vi "Error Dialog.vi"(6 "Modal (T)":bool=TRUE, 8 "error in (no error)":errorcluster) -> (0 "error out":errorcluster)   [LabVIEW 2017, in "Error Dialog w Copy to Clipboard.lvlib"]
doc: "Displays error message to the user.\n\nCopyright (c) 2022, Neosoft Technologies Inc\nAll rights reserved."
uses:
  Error Dialog w Copy to Clipboard.lvlib
  <vilib>/Utility/error.llb/DialogType.ctl
  <vilib>/Platform/browser.llb/Open URL in Default Browser (string).vi
panel:
  out "String":string
  out "Error Code":string
  in  "Show details":bool
  in  "Google":bool
  in  "Copy":bool
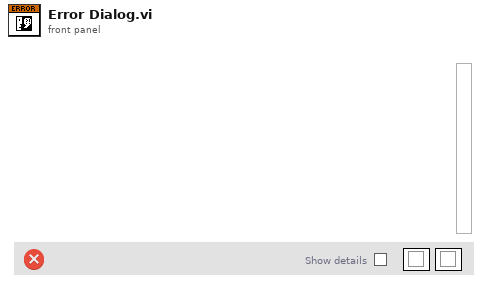
[diagram p1: front panel]
types:
  T1 = enum32{"Invalid", "Default", "Floating", "Floating/Auto-Hide", "Modal"}
  T2 = enum32{"Invalid", "Standard", "Closed", "Hidden", "Minimized", "Maximized"}
  T3 = cluster{"call chain":string[], "error":errorcluster, "show details":bool, "message":string}
  T4 = typedef "DialogType.ctl" = u16
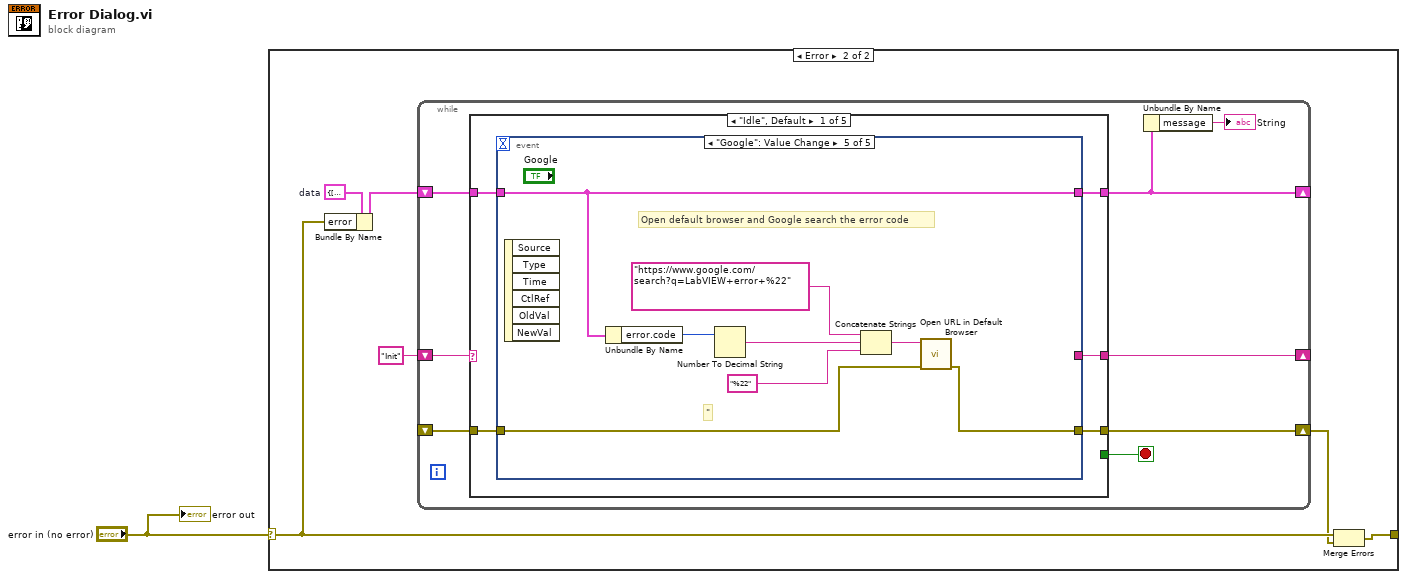
[diagram p0: block diagram]
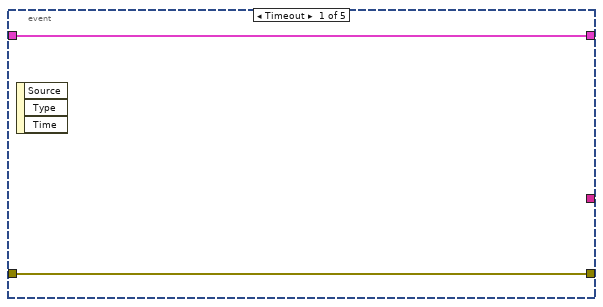
[diagram p3: hidden frame]
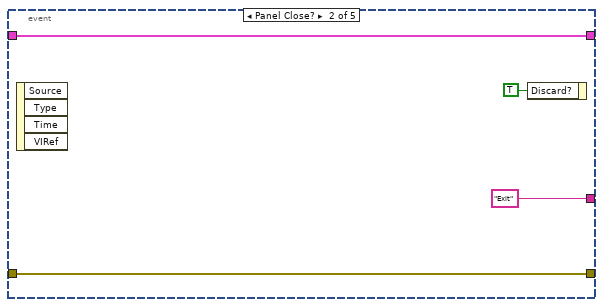
[diagram p4: hidden frame]
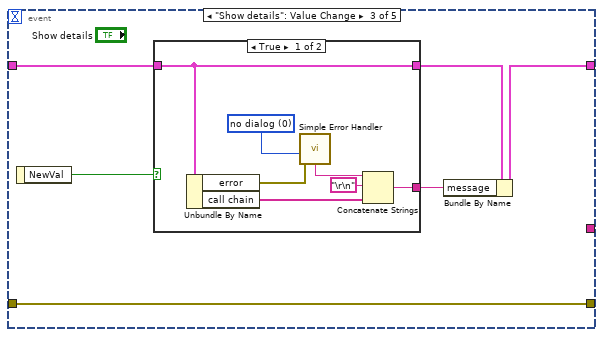
[diagram p5: hidden frame]
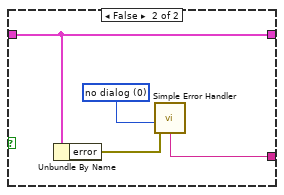
[diagram p6: hidden frame]
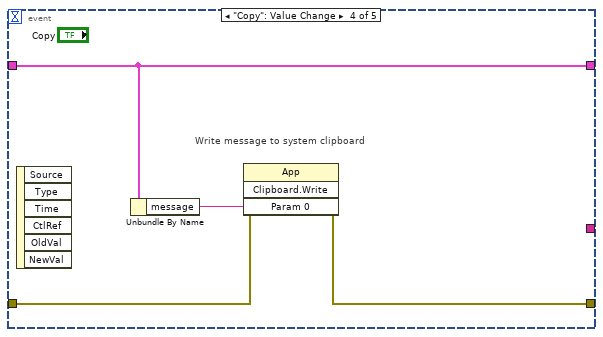
[diagram p7: hidden frame]
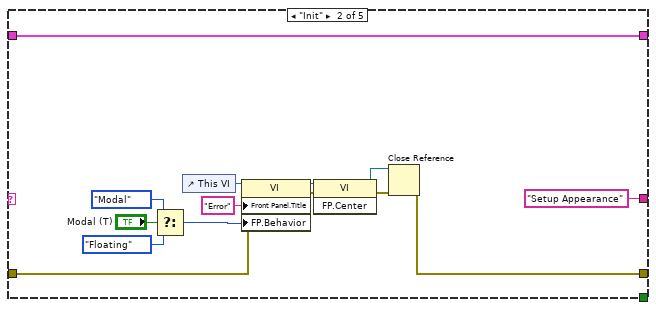
[diagram p8: hidden frame]
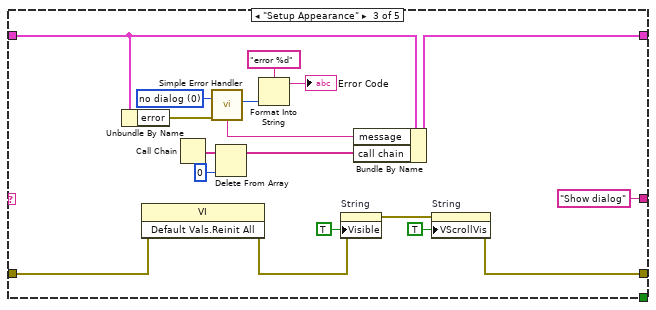
[diagram p9: hidden frame]
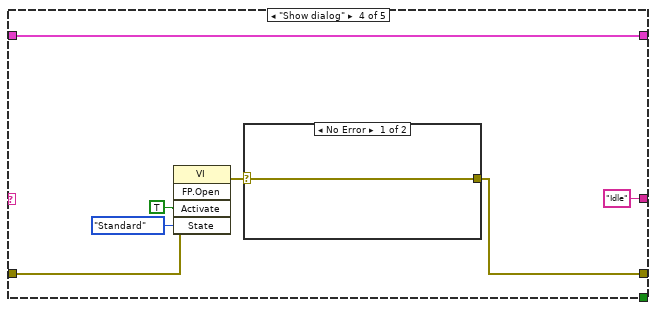
[diagram p10: hidden frame]
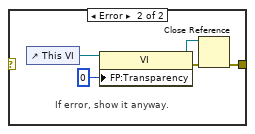
[diagram p11: hidden frame]
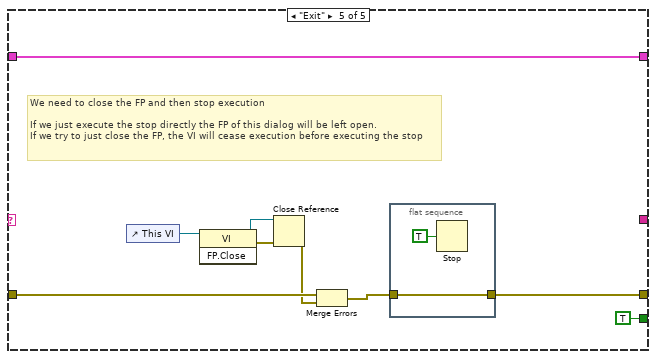
[diagram p12: hidden frame]
diagram:
  n1 = case shown="Error" "error in (no error)" {
    selector: "error in (no error)" -> [w2 w5]
    tunnel: [w2 w4] -> _
    frame No Error {
    }
    frame Error {
      w7 = T3 {"call chain"=[], "error"={"status"=FALSE, "code"=0, "source"=""}, "show details"=FALSE, "message"=""}  # data
      n2 = Bundle By Name(cluster=w7, "error"=w5) -> (w6:T3)
      n3 = while {
        shift-right: [w14] -> _
        shift-left: "Init" ("format string") -> [w15]
        shift-right: [w13] -> w3
        shift-left: _ -> [w12]
        shift-right: [w10] -> _
        shift-left: w6 -> [w11]
        stop <- w16 stop-if-true
        n4 = case shown="\"Idle\", Default" w15 {
          tunnel: [_ _ _ _ TRUE ("Discard?")] -> w16
          tunnel: [w17 "Setup Appearance" "Show dialog" "Idle" _] -> w14
          tunnel: [w20 w63 w79 w89 w104] -> w13
          tunnel: w12 -> [w21 w62 w72 w90 w110]
          tunnel: [w18 w61 w78 w95 w103] -> w10
          tunnel: w11 -> [w19 w61 w87 w95 w103]
          frame "Idle", Default {
            n5 = event shown="[4] \"Google\": Value Change" {
              selector: _ -> [_ _ _ _ _]
              dyn-events: _ -> [_ _ _ _ _]
              timeout: _ -> [_ _ _ _ _]
              tunnel: w21 -> [w23 w27 w33 w46 w54]
              tunnel: [w23 w27 w33 w45 w53] -> w20
              tunnel: w19 -> [w22 w26 w31 w48 w56]
              tunnel: [w22 w26 w29 w48 w56] -> w18
              tunnel: [_ "Exit" ("format string") _ _ _] -> w17
              event Timeout {
                n6 = event-data() -> ()  [unwired: 1 in, 3 out]
              }
              event Panel Close? {
                n7 = event-data() -> ()  [unwired: 1 in, 4 out]
                n8 = event-data("Discard?"=TRUE) -> ()  [unwired: 1 in, 1 out]
              }
              event "Show details": Value Change {
                n9 = event-data() -> ("NewVal"=w32:bool)  [unwired: 1 in]
                n10 = case shown="True" w32 {
                  tunnel: w31 -> [w38 w42]
                  tunnel: [w38 w42] -> w30
                  tunnel: [w34 w41] -> w28
                  frame True {
                    w37 = "\r\n"
                    w40 = T4 0 items=["no dialog", "OK message", "continue or stop message", "OK message + warnings", "continue/stop + warnings"] ("type of dialog (OK msg:1)")
                    n11 = Unbundle By Name(w38) -> ("error"=w39:errorcluster, "call chain"=w35:string[])
                    n12 = call <vilib>:"Simple Error Handler.vi"("type of dialog (OK msg:1)"=w40, "error in (no error)"=w39) -> ("message"=w36:string)  [unwired: 3 in, 4 out]
                    n13 = Concatenate Strings(w36, w37, w37, w35) -> (w34:string)
                  }
                  frame False {
                    w44 = T4 0 items=["no dialog", "OK message", "continue or stop message", "OK message + warnings", "continue/stop + warnings"] ("type of dialog (OK msg:1)")
                    n14 = Unbundle By Name(w42) -> ("error"=w43:errorcluster)
                    n15 = call <vilib>:"Simple Error Handler.vi"("type of dialog (OK msg:1)"=w44, "error in (no error)"=w43) -> ("message"=w41:string)  [unwired: 3 in, 4 out]
                  }
                }
                n16 = Bundle By Name(cluster=w30, "message"=w28) -> (w29:T3)
              }
              event "Copy": Value Change {
                # "Write message to system clipboard"
                n17 = event-data() -> ()  [unwired: 1 in, 6 out]
                n18 = Unbundle By Name(w48) -> ("message"=w47:string)
                n19 = invoke class="App" method="Clipboard.Write"(error in=w46, "Param 0"=w47) -> (error out=w45:errorcluster)  [unwired: 2 in, 3 out]
              }
              event "Google": Value Change {
                # "\""
                # "Open default browser and Google search the error code"
                n20 = event-data() -> ()  [unwired: 1 in, 6 out]
                n21 = Unbundle By Name(w56) -> ("error.code"=w50:i32)
                n22 = Number To Decimal String(number=w50) -> (decimal integer string=w49:string)  [unwired: 1 in]
                n23 = Concatenate Strings("https://www.google.com/search?q=LabVIEW+error+%22" ("format string"), w49, "%22") -> (w52:string)
                n24 = call-poly <vilib>:"Open URL in Default Browser.vi"("error in (no error)"=w54, "URL"=w52) -> ("error out"=w53:errorcluster)  [unwired: 4 in, 1 out]
              }
            }
          }
          frame "Init" {
            n25 = Select(t=T1."Modal" ("Front Panel Window:Behavior"), s="Modal (T)", f=T1."Floating") -> (s? t:f=w57:T1)
            n26 = control-ref of="This VI"() -> (w68:refnum<vi>)
            n27 = property class="VI"(reference=w68, error in=w62, "Front Panel.Title"="Error" ("Front Panel Window:Title"), "FP.Behavior"=w57) -> (reference out=w69:refnum<vi>, error out=w70:errorcluster)
            n28 = invoke class="VI" method="FP.Center"(reference=w69, error in=w70) -> (reference out=w66:refnum<vi>, error out=w65:errorcluster)  [unwired: 1 in, 1 out]
            n29 = Close Reference(reference=w66, error in (no error)=w65) -> (error out=w63:errorcluster)
          }
          frame "Setup Appearance" {
            w85 = T4 0 items=["no dialog", "OK message", "continue or stop message", "OK message + warnings", "continue/stop + warnings"] ("type of dialog (OK msg:1)")
            n30 = Unbundle By Name(w87) -> ("error"=w86:errorcluster)
            n31 = invoke class="VI" method="Default Vals.Reinit All"(error in=w72) -> (error out=w71:errorcluster)  [unwired: 2 in, 2 out]
            n32 = Call Chain() -> (call chain=w75:string[])
            n33 = call <vilib>:"Simple Error Handler.vi"("type of dialog (OK msg:1)"=w85, "error in (no error)"=w86) -> ("code out"=w84:i32, "message"=w77:string)  [unwired: 3 in, 3 out]
            n34 = Delete From Array(array=w75, index=0) -> (array with subset deleted=w74:string[])  [unwired: 1 in, 1 out]
            n35 = Format Into String(format string="error %d", w84) -> (resulting string=→"Error Code":string)  [unwired: 2 in, 1 out]
            n36 = property on="String" class="Str"(error in=w71, "Visible"=TRUE) -> (error out=w81:errorcluster)  [unwired: 1 in, 1 out]
            n37 = Bundle By Name(cluster=w87, "message"=w77, "call chain"=w74) -> (w78:T3)
            n38 = property on="String" class="Str"(error in=w81, "VScrollVis"=TRUE ("Vertical Scrollbar Visible")) -> (error out=w79:errorcluster)  [unwired: 1 in, 1 out]
          }
          frame "Show dialog" {
            n39 = invoke class="VI" method="FP.Open"(error in=w90, "Activate"=TRUE ("Front Panel Window:Open"), "State"=T2."Standard") -> (error out=w93:errorcluster)  [unwired: 2 in, 4 out]
            n40 = case shown="No Error" w93 {
              selector: w93 -> [w96 _]
              tunnel: [w96 w97] -> w89
              frame No Error {
              }
              frame Error {
                # "If error, show it anyway."
                n41 = control-ref of="This VI"() -> (w99:refnum<vi>)
                n42 = property class="VI"(reference=w99, "FP:Transparency"=u8 0 ("Front Panel Window:Transparency")) -> (reference out=w100:refnum<vi>, error out=w101:errorcluster)  [unwired: 1 in]
                n43 = Close Reference(reference=w100, error in (no error)=w101) -> (error out=w97:errorcluster)
              }
            }
          }
          frame "Exit" {
            # "We need to close the FP and then stop execution\n\nIf we just execute the stop directly the FP of this dialog will be left open.\nIf we try to just close the FP, the VI will cease execution before executing the stop"
            n44 = control-ref of="This VI"() -> (w108:refnum<vi>)
            n45 = invoke class="VI" method="FP.Close"(reference=w108) -> (reference out=w106:refnum<vi>, error out=w107:errorcluster)  [unwired: 2 in, 1 out]
            n46 = Close Reference(reference=w106, error in (no error)=w107) -> (error out=w105:errorcluster)
            n47 = Merge Errors(w110, w105) -> (w102:errorcluster)
            n48 = flat-sequence {
              tunnel: w102 -> [w111]
              tunnel: [w111] -> w104
              frame #0 {
                n49 = Stop(stop? (T)=TRUE) -> ()
              }
            }
          }
        }
        n50 = Unbundle By Name(w10) -> ("message"=→"String":string)
      }
      n51 = Merge Errors(w5, w3) -> (w4:errorcluster)
    }
  }
  "error out" <- "error in (no error)"
